vi "Write Transfer Group Buffer.vi"(8 "error in":errorcluster, 9 "data":string, 10 "Transfer Group":refnum<class "Transfer Group.lvclass">, 11 "RDMA Transceiver in":refnum<class "RDMA Transceiver.lvclass">) -> (0 "error out":errorcluster, 3 "RDMA Transceiver out":refnum<class "RDMA Transceiver.lvclass">)   [LabVIEW 2020, in "RDMA.lvlib" / "RDMA Transceiver.lvclass"]
uses:
  RDMA Transceiver.lvclass
  RDMA Transceiver.lvclass/RDMA Transceiver.ctl
  Throw Size Mismatch Error.vi
  DSF Core.lvlibp/Classes/Transfer Group/Transfer Group.lvclass
  DSF Core.lvlibp/Classes/Buffer/Buffer.lvclass
  DSF Core.lvlibp/Classes/Buffer/Write Buffer 1D U8.vi
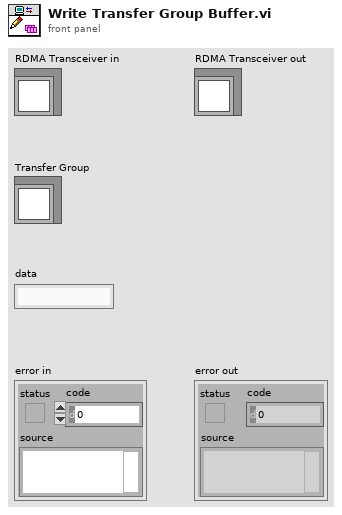
[diagram p1: front panel]
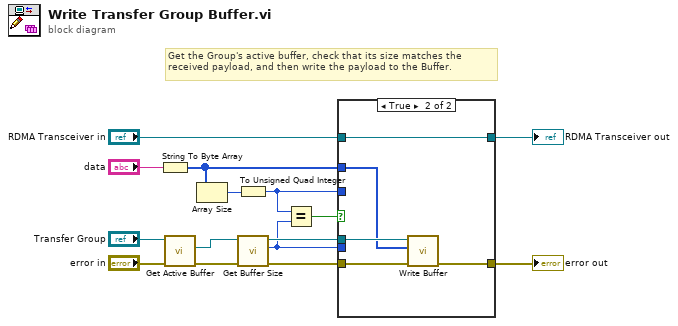
[diagram p0: block diagram]
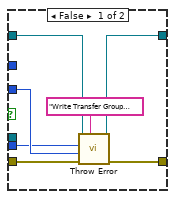
[diagram p2: hidden frame]
diagram:
  # "Get the Group's active buffer, check that its size matches the received payload, and then write the payload to the Buffer."
  n1 = String To Byte Array(string="data") -> (unsigned byte array=w12:u8[])
  n2 = call "Get Active Buffer.vi"("error in (no error)"="error in", "Transfer Group in"="Transfer Group") -> ("error out"=w2:errorcluster, "Buffer"=w1:refnum<class "Buffer.lvclass">)  [unwired: 7 in, 1 out]
  n3 = Array Size(array=w12) -> (size(s)=w14:i32)
  n4 = To Unsigned Quad Integer(1:w14) -> (0:w9:u64)
  n5 = call "Get Buffer Size.vi"("Buffer in"=w1) -> ("buffer size"=w10:u64, "Buffer out"=w13:refnum<class "Buffer.lvclass">)  [unwired: 9 in]
  n6 = Equal?(x=w9, y=w10) -> (x = y?=w11:bool)
  n7 = case shown="True" w11 {
    tunnel: w13 -> [_ w26]
    tunnel: w2 -> [w21 w25]
    tunnel: [w20 w24] -> w8
    tunnel: w12 -> [_ w22]
    tunnel: "RDMA Transceiver in" -> [w19 w23]
    tunnel: [w18 w23] -> w7
    tunnel: w10 -> [w16 _]
    tunnel: w9 -> [w17 _]
    frame False {
      n8 = call-poly "Throw Error.vi"("source vi name"="Write Transfer Group Buffer", "error in"=w21, "actual size"=w17, "expected size"=w16, "RDMA in"=w19) -> ("error out"=w20:errorcluster, "RDMA out"=w18:refnum<class "RDMA Transceiver.lvclass">)  [unwired: 5 in]
    }
    frame True {
      n9 = call-poly "Write Buffer.vi"("error in (no error)"=w25, "src array in"=w22, "Buffer in"=w26) -> ("error out"=w24:errorcluster)  [unwired: 5 in, 3 out]
    }
  }
  "error out" <- w8
  "RDMA Transceiver out" <- w7
